vi "OceanOpticsReadOut.vi"() -> ()   [LabVIEW 2015]
uses:
  C:/Program Files/Ocean Optics/OmniDriver/OOI_HOME/OmniDriver32.dll
  C:/Program Files/Ocean Optics/OmniDriver/OOI_HOME/common32.dll
panel:
  in  "stop":bool
  out "Last Exception":string
  out "Spectrum":cluster{"X":dbl, "Y":dbl}[](graph)
  out "Spectrum Values":dbl[](array[numeric])
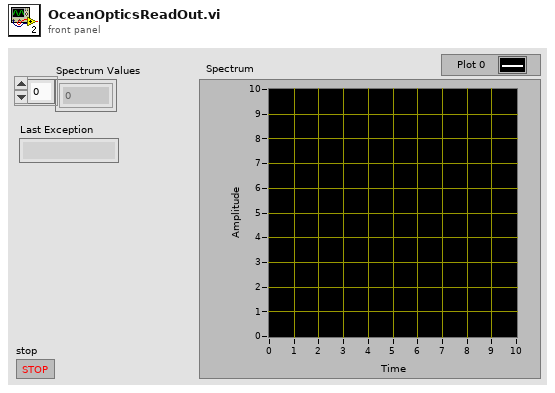
[diagram p1: front panel]
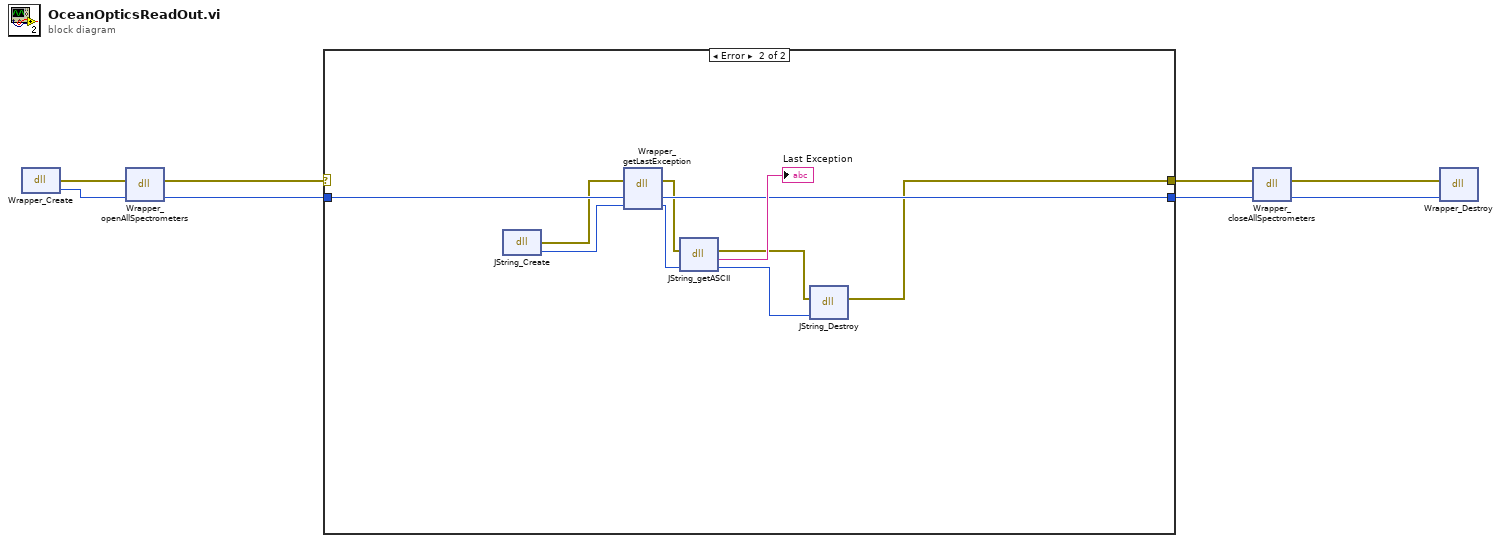
[diagram p0: block diagram]
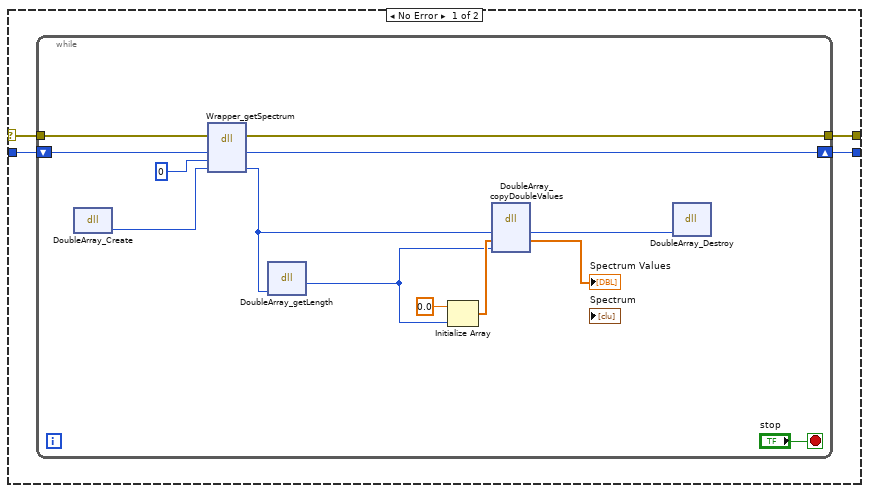
[diagram p2: hidden frame]
diagram:
  n1 = dll-call lib="C:/Program Files/Ocean Optics/OmniDriver/OOI_HOME/OmniDriver32.dll" fn="Wrapper_Create" label="Wrapper.Create"() -> (error out=w7:errorcluster, "return type"=w8:u32)  [unwired: 3 in, 1 out]
  n2 = dll-call lib="C:/Program Files/Ocean Optics/OmniDriver/OOI_HOME/OmniDriver32.dll" fn="Wrapper_openAllSpectrometers" label="Wrapper.openAllSpectrometers"(error in=w7, "Wrapper"=w8) -> (error out=w6:errorcluster, "Wrapper"=w5:u32)  [unwired: 2 in, 2 out]
  n3 = case shown="Error" w6 {
    selector: w6 -> [w9 _]
    tunnel: w5 -> [w12 w31]
    tunnel: [w11 w30] -> w2
    tunnel: [w10 w26] -> w1
    frame No Error {
      n4 = while {
        shift-right: [w19] -> w11
        shift-left: w12 -> [w18]
        tunnel: w9 -> [w21]
        tunnel: [w20] -> w10
        stop <- "stop" stop-if-true
        n5 = dll-call lib="C:/Program Files/Ocean Optics/OmniDriver/OOI_HOME/common32.dll" fn="DoubleArray_Create" label="DoubleArray.Create"() -> ("return type"=w16:u32)  [unwired: 3 in, 2 out]
        n6 = dll-call lib="C:/Program Files/Ocean Optics/OmniDriver/OOI_HOME/OmniDriver32.dll" fn="Wrapper_getSpectrum" label="Wrapper.getSpectrum"(error in=w21, "Wrapper"=w18, "Index"=0, "DoubbleArray"=w16) -> (error out=w20:errorcluster, "Wrapper"=w19:u32, "DoubbleArray"=w15:u32)  [unwired: 3 in, 2 out]
        n7 = dll-call lib="C:/Program Files/Ocean Optics/OmniDriver/OOI_HOME/common32.dll" fn="DoubleArray_getLength" label="DoubleArray.getLength"("DoubleArray"=w15) -> ("return type"=w14:i32)  [unwired: 4 in, 2 out]
        n8 = Initialize Array(0.0 ("element"), w14) -> (w22:dbl[])
        n9 = dll-call lib="C:/Program Files/Ocean Optics/OmniDriver/OOI_HOME/common32.dll" fn="DoubleArray_copyDoubleValues" label="DoubleArray.copyDoubleValues"("DoubbleArray"=w15, "Values"=w22, "Length"=w14) -> ("DoubbleArray"=w24:u32, "Values"=→"Spectrum Values":dbl[])  [unwired: 4 in, 3 out]
        n10 = dll-call lib="C:/Program Files/Ocean Optics/OmniDriver/OOI_HOME/common32.dll" fn="DoubleArray_Destroy" label="DoubleArray.Destroy"("DoubleArray"=w24) -> ()  [unwired: 4 in, 3 out]
      }
    }
    frame Error {
      n11 = dll-call lib="C:/Program Files/Ocean Optics/OmniDriver/OOI_HOME/common32.dll" fn="JString_Create" label="JString.Create"() -> (error out=w29:errorcluster, "return type"=w35:u32)  [unwired: 3 in, 1 out]
      n12 = dll-call lib="C:/Program Files/Ocean Optics/OmniDriver/OOI_HOME/OmniDriver32.dll" fn="Wrapper_getLastException" label="Wrapper.getLastException"(error in=w29, "Wrapper"=w31, "Exception JString"=w35) -> (error out=w28:errorcluster, "Wrapper"=w30:u32, "Exception JString"=w34:u32)  [unwired: 2 in, 2 out]
      n13 = dll-call lib="C:/Program Files/Ocean Optics/OmniDriver/OOI_HOME/common32.dll" fn="JString_getASCII" label="JString.getASCII"(error in=w28, "JString"=w34) -> (error out=w27:errorcluster, "return type"=→"Last Exception":string, "JString"=w33:u32)  [unwired: 2 in, 1 out]
      n14 = dll-call lib="C:/Program Files/Ocean Optics/OmniDriver/OOI_HOME/common32.dll" fn="JString_Destroy" label="JString.Destroy"(error in=w27, "JString"=w33) -> (error out=w26:errorcluster)  [unwired: 3 in, 2 out]
    }
  }
  n15 = dll-call lib="C:/Program Files/Ocean Optics/OmniDriver/OOI_HOME/OmniDriver32.dll" fn="Wrapper_closeAllSpectrometers" label="Wrapper.closeAllSpectrometers"(error in=w1, "Wrapper"=w2) -> (error out=w4:errorcluster, "Wrapper"=w3:u32)  [unwired: 2 in, 2 out]
  n16 = dll-call lib="C:/Program Files/Ocean Optics/OmniDriver/OOI_HOME/OmniDriver32.dll" fn="Wrapper_Destroy" label="Wrapper.Destroy"(error in=w4, "Wrapper"=w3) -> ()  [unwired: 3 in, 3 out]
